vi "Kelvinox_Parse_Heater_Excitation_to_Number.vi"(1 "Excitation String":string) -> (0 "Excitation Level":dbl)   [LabVIEW 2019]
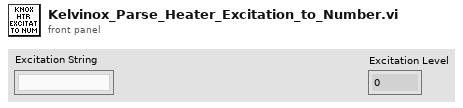
[diagram p1: front panel]
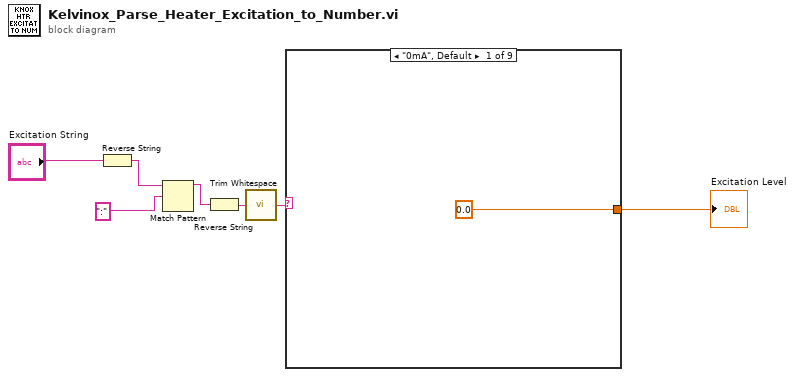
[diagram p0: block diagram]
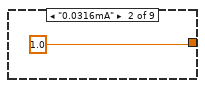
[diagram p2: hidden frame]
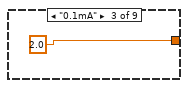
[diagram p3: hidden frame]
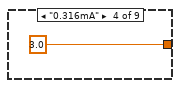
[diagram p4: hidden frame]
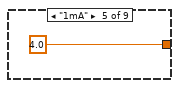
[diagram p5: hidden frame]
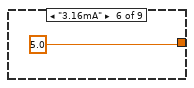
[diagram p6: hidden frame]
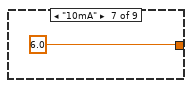
[diagram p7: hidden frame]
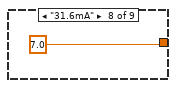
[diagram p8: hidden frame]
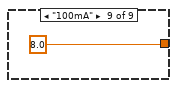
[diagram p9: hidden frame]
diagram:
  n1 = Reverse String(1:"Excitation String") -> (0:w6:string)
  n2 = Match Pattern(string=w6, regular expression=":") -> (before substring=w4:string)  [unwired: 1 in, 3 out]
  n3 = Reverse String(1:w4) -> (0:w2:string)
  n4 = call <vilib>:"Trim Whitespace.vi"("string"=w2) -> ("trimmed string"=w1:string)  [unwired: 1 in]
  n5 = case shown="\"0mA\", Default" w1 {
    tunnel: [0.0 1.0 2.0 3.0 4.0 5.0 6.0 7.0 8.0] -> w7
    frame "0mA", Default {
    }
    frame "0.0316mA" {
    }
    frame "0.1mA" {
    }
    frame "0.316mA" {
    }
    frame "1mA" {
    }
    frame "3.16mA" {
    }
    frame "10mA" {
    }
    frame "31.6mA" {
    }
    frame "100mA" {
    }
  }
  "Excitation Level" <- w7
